vi "Example Math 2.vi"() -> ()   [LabVIEW 2014]
uses:
  <vilib>/LabVIEW Universal Transcriptor/Arduino for LabVIEW Complex numbers/Complex Numbers.lvlib
panel:
  out "Error Out":errorcluster
  in  "Error In":errorcluster
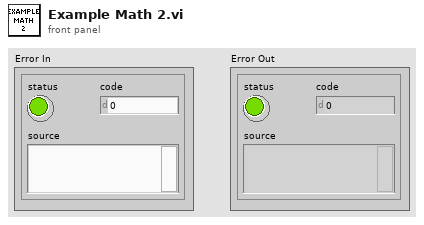
[diagram p1: front panel]
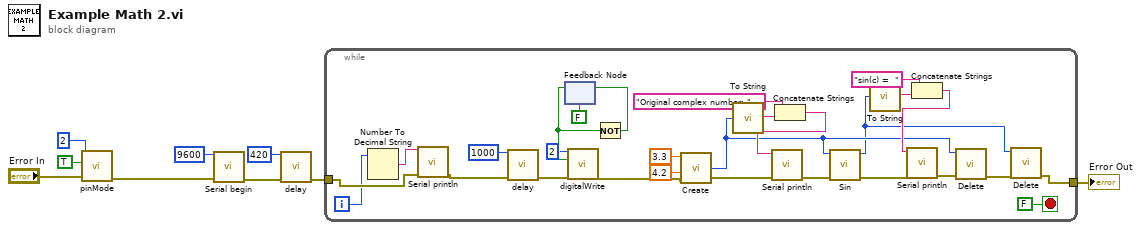
[diagram p0: block diagram]
diagram:
  n1 = call "pinMode.vi"("Error In"="Error In", "output?"=TRUE, "pin number"=2) -> ("Error Out"=w2:errorcluster)  [unwired: 8 in]
  n2 = call "Serial begin.vi"("Error In"=w2, "speed (Bd)"=9600) -> ("Error Out"=w8:errorcluster)  [unwired: 9 in]
  n3 = call "delay.vi"("Error In"=w8, "time (ms)"=420) -> ("Error Out"=w6:errorcluster)  [unwired: 9 in]
  n4 = while {
    tunnel: w6 -> [w35]
    tunnel: [w12] -> w1
    i -> [w28]
    stop <- FALSE stop-if-true
    n5 = Number To Decimal String(number=w28) -> (decimal integer string=w36:string)  [unwired: 1 in]
    n6 = call "Serial println.vi"("Error In"=w35, "string in"=w36) -> ("Error Out"=w33:errorcluster)  [unwired: 9 in]
    n7 = call "delay.vi"("Error In"=w33, "time (ms)"=1000) -> ("Error Out"=w32:errorcluster)  [unwired: 9 in]
    n8 = feedback #1(FALSE) -> (w30:bool)
    n9 = call "digitalWrite.vi"("Error In"=w32, "value"=w30, "pin number"=2) -> ("Error Out"=w26:errorcluster)  [unwired: 8 in]
    n10 = Not(x=w30) -> (.not. x?=w27:bool)
    n11 = feedback-in #1(w27) -> ()
    n12 = call <vilib>:"Create.vi"("Error In"=w26, "Imag"=4.2, "Real"=3.3) -> ("Error Out"=w20:errorcluster, "Complex"=w11:u32)  [unwired: 2 in]
    n13 = call <vilib>:"To String.vi"("Complex number"=w11) -> ("String complex num."=w23:string)
    n14 = Concatenate Strings("Original complex number: " ("string"), w23) -> (w21:string)
    n15 = call "Serial println.vi"("Error In"=w20, "string in"=w21) -> ("Error Out"=w19:errorcluster)  [unwired: 9 in]
    n16 = call <vilib>:"Sin.vi"("Error In"=w19, "A"=w11) -> ("Error Out"=w16:errorcluster, "sin(A)"=w10:u32)  [unwired: 8 in]
    n17 = call <vilib>:"To String.vi"("Complex number"=w10) -> ("String complex num."=w17:string)
    n18 = Concatenate Strings("sin(c) =  " ("string"), w17) -> (w15:string)
    n19 = call "Serial println.vi"("Error In"=w16, "string in"=w15) -> ("Error Out"=w14:errorcluster)  [unwired: 9 in]
    n20 = call <vilib>:"Delete.vi"("Error In"=w14, "Numeric"=w11) -> ("Error Out"=w13:errorcluster)  [unwired: 9 in]
    n21 = call <vilib>:"Delete.vi"("Error In"=w13, "Numeric"=w10) -> ("Error Out"=w12:errorcluster)  [unwired: 9 in]
  }
  "Error Out" <- w1
